vi "Parse Field Cardinality.vi"(6 "Field in":T1={"Name"="", "Number"=0, "Optional"=FALSE, "Repeated"=FALSE, "Type"={"Type"=enum."double", "Subtype"=""}, "Key Type"={"Type"=enum."double", "Subtype"=""}, "Value Type"={"Type"=enum."double", "Subtype"=""}}, 8 "error in (no error)":errorcluster, 10 "Text":string, 11 "ProtoParser in":refnum<class "ProtoParser.lvclass">) -> (0 "error out":errorcluster, 2 "Remaining":string, 3 "ProtoParser out":refnum<class "ProtoParser.lvclass">, 4 "Field":T1={"Name"="", "Number"=0, "Optional"=FALSE, "Repeated"=FALSE, "Type"={"Type"=enum."double", "Subtype"=""}, "Key Type"={"Type"=enum."double", "Subtype"=""}, "Value Type"={"Type"=enum."double", "Subtype"=""}})   [LabVIEW 2020, in "LV-Protoc.lvlib" / "ProtoParser.lvclass"]
uses:
  ProtoParser.lvclass
  LV-Proto/Field.ctl
  LV-Proto/Type.ctl
  LV-Proto/Proto Type.ctl
  LV-Proto/LV-Proto.lvlib
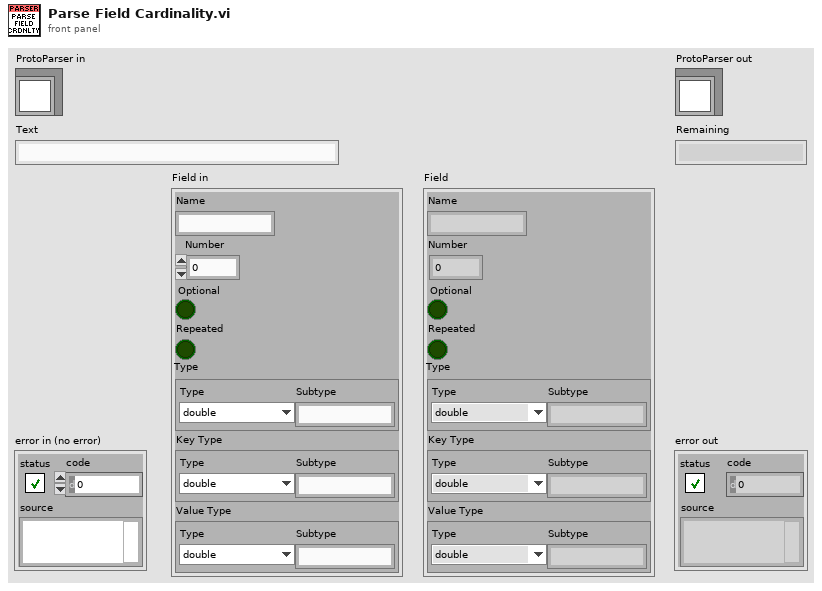
[diagram p1: front panel]
types:
  T1 = typedef "LV-Proto.lvlib/Field.ctl" = cluster{"Name":string, "Number":u32, "Optional":bool, "Repeated":bool, "Type":T2, "Key Type":T2, "Value Type":T2}
  T2 = typedef "LV-Proto.lvlib/Type.ctl" = cluster{"Type":T3, "Subtype":string}
  T3 = typedef "LV-Proto.lvlib/Proto Type.ctl" = enum16{"UNKNOWN", "double", "float", "int32", "int64", "uint32", "uint64", "sint32", "sint64", "fixed32", "fixed64", "sfixed32", "sfixed64", "bool", "string", "bytes", "enum", "map", "message"}
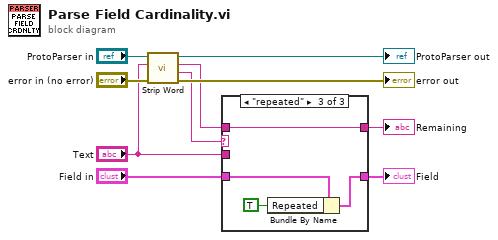
[diagram p0: block diagram]
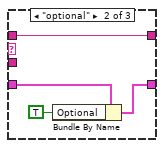
[diagram p3: hidden frame]
diagram:
  n1 = call "Strip Word.vi"("error in (no error)"="error in (no error)", "String"="Text", "ProtoParser in"="ProtoParser in") -> ("error out"=→"error out":errorcluster, "Word"=w7:string, "Remaining"=w5:string, "ProtoParser out"=→"ProtoParser out":refnum<class "ProtoParser.lvclass">)  [unwired: 5 in]
  n2 = case shown="\"repeated\"" w7 {
    tunnel: "Field in" -> [w12 w16 w20]
    tunnel: w5 -> [_ w13 w17]
    tunnel: "Text" -> [w11 _ _]
    tunnel: [w12 w14 w18] -> w2
    tunnel: [w11 w13 w17] -> w1
    frame Default {
    }
    frame "optional" {
      n3 = Bundle By Name(cluster=w16, "Optional"=TRUE) -> (w14:T1)
    }
    frame "repeated" {
      n4 = Bundle By Name(cluster=w20, "Repeated"=TRUE) -> (w18:T1)
    }
  }
  "Remaining" <- w1
  "Field" <- w2
